vi "oax_gsSet SubVI Control Value.vi"(1 "Boolean":bool, 2 "vi reference in":refnum<vi>) -> (0 "vi reference out":refnum<vi>)   [LabVIEW 2017]
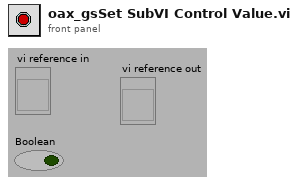
[diagram p1: front panel]
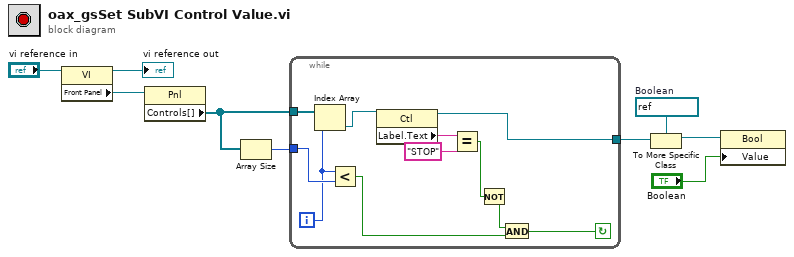
[diagram p0: block diagram]
diagram:
  w3 = refnum<vi> refnum  # Boolean
  n1 = property class="VI"(reference="vi reference in") -> (reference out=→"vi reference out":refnum<vi>, "Front Panel"=w9:refnum<vi>)  [unwired: 1 in, 1 out]
  n2 = property class="Pnl"(reference=w9) -> ("Controls[]"=w7:refnum<vi>[])  [unwired: 1 in, 2 out]
  n3 = Array Size(array=w7) -> (size(s)=w6:i32)
  n4 = while {
    tunnel: w7 -> [w18]
    tunnel: w6 -> [w16]
    tunnel: [w10] -> w5
    i -> [w15]
    stop <- w13 continue-if-true
    n5 = Index Array(array=w18, index=w15) -> (element=w17:refnum<vi>)
    n6 = Less?(x=w15, y=w16) -> (x < y?=w14:bool)
    n7 = property class="Ctl"(reference=w17) -> (reference out=w10:refnum<vi>, "Label.Text"=w20:string)  [unwired: 1 in, 1 out]
    n8 = Equal?(x=w20, y="STOP") -> (x = y?=w11:bool)
    n9 = Not(x=w11) -> (.not. x?=w12:bool)
    n10 = And(x=w12, y=w14) -> (x .and. y?=w13:bool)
  }
  n11 = To More Specific Class(target class=w3, reference=w5) -> (specific class reference=w4:refnum<vi>)  [unwired: 1 in, 1 out]
  n12 = property class="Bool"(reference=w4, "Value"="Boolean") -> ()  [unwired: 1 in, 2 out]
